vi "DelayPtsAdjust.vi"(7 "CalcPt?":bool=TRUE, 10 "Digitizer Settings":T1 {"Trigger Settings"."Trig Slope" items=["Positive", "Negative"]; "Trigger Settings"."Level (mV)" format="%.2f"; "Trigger Settings"."Trig Coupling" items=["DC 1 MOhm", "AC 1 MOhm", "DC 50 Ohm", "AC 50 Ohm"]; "Trigger Settings"."Trig Source" items=["Chan 1", "External"]; "Rel Dig Delay" format="%.2f"; "DigTimeOut" format="%.2f"; "Avg Num" min=1; "Offset delay (us)" format="%.2f"; "Additional dig delay (us)" format="%.2f"; "Digitizer delay (us)" format="%.2f"}, 11 "Delay in Pts":u32) -> (2 "Actual Delay pts":u32, 3 "PostDelayCorrection":u32)   [LabVIEW 2022 SP3]
uses:
  DigitizerSettings.ctl
  Digitizer.ctl
  DigConfig.ctl
  DigitizerID.ctl
  C:/Windows/System32/ADQAPI_dotNet_helper.dll
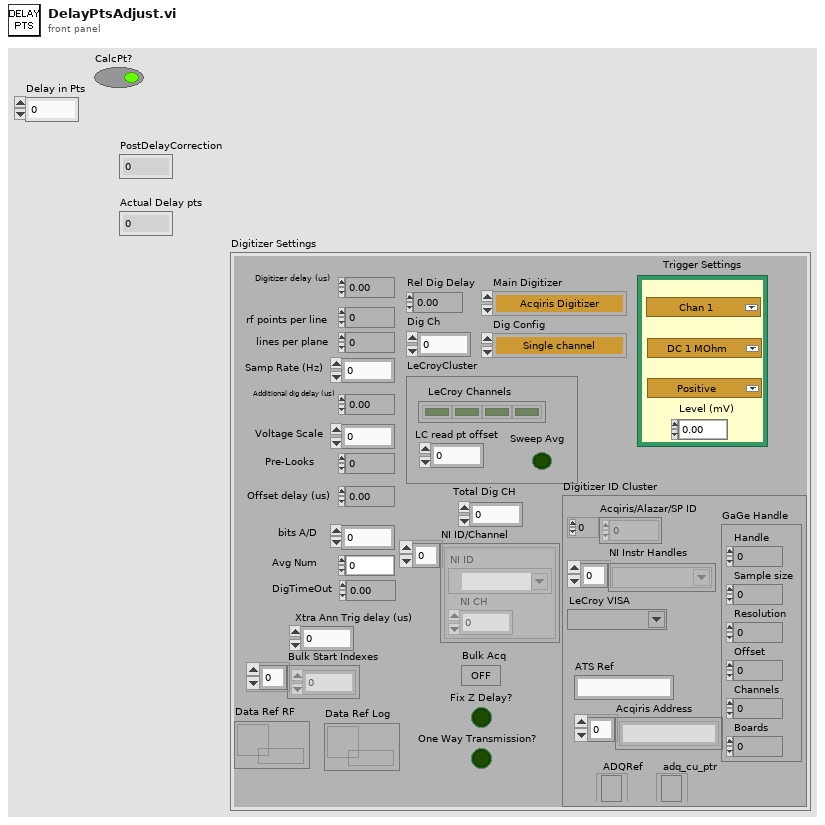
[diagram p1: front panel]
types:
  T1 = typedef "DigitizerSettings.ctl" = cluster{"Digitizer delay (us) ":dbl, "rf points per line":i32, "lines per plane":i32, "Samp Rate (Hz)":dbl, "Additional dig delay (us)":dbl, "Voltage Scale":dbl, "Pre-Looks":i32, "Offset delay (us)":dbl, "bits A/D":i8, "Avg Num":i32, "DigTimeOut":sgl, "Rel Dig Delay":sgl, "Dig Ch":i32, "LeCroyCluster":cluster{"LeCroy Channels":bool[], "LC read pt offset":dbl, "Sweep Avg":bool}, "Main Digitizer":T2, "Dig Config":T3, "Digitizer ID Cluster":T4, "Trigger Settings":cluster{"Trig Source":u16, "Trig Coupling":u16, "Trig Slope":u16, "Level (mV)":dbl}, "Bulk Acq":bool, "Bulk Start Indexes":i32[], "Data Ref RF":refnum<data-value>, "NI ID/Channel":cluster{"NI ID":refnum<k15>, "NI CH":i32}[], "Total Dig CH":i32, "Xtra Ann Trig delay (us)":dbl, "Fix Z Delay?":bool, "One Way Transmission?":bool, "Data Ref Log":refnum<data-value>}
  T2 = typedef "Digitizer.ctl" = enum16{"Acqiris Digitizer", "NI Digitizer", "LeCroy", "GaGe", "AlazarTech", "No Digitizer", "Teledyne"}
  T3 = typedef "DigConfig.ctl" = enum16{"Single channel", "2 Chans w/ 2 Acqiris", "2 Chans w/ 1 Acqiris", "5-CH Pulser New", "5-CH pulser w/ ann array", "5-pass style ann array", "Empty"}
  T4 = typedef "DigitizerID.ctl" = cluster{"Acqiris/Alazar/SP ID":u32[], "NI Instr Handles":refnum<k15>[], "LeCroy VISA":refnum<visa-resource-name>, "GaGe Handle":cluster{"Handle":u32, "Sample size":u32, "Resolution":i32, "Offset":i32, "Channels":u32, "Boards":u32}, "ATS Ref":string, "Acqiris Address":string[], "ADQRef":refnum<k24>, "adq_cu_ptr":refnum<k24>}
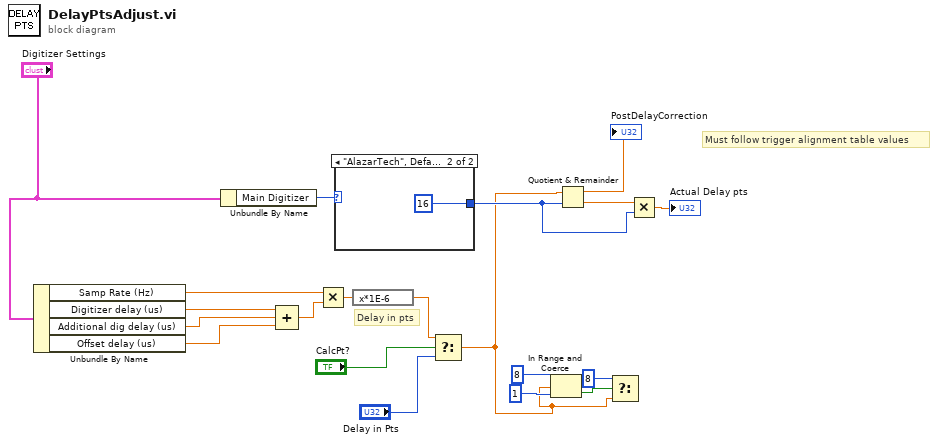
[diagram p0: block diagram]
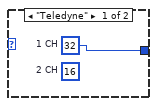
[diagram p2: hidden frame]
diagram:
  # "Delay in pts"
  # "Must follow trigger alignment table values"
  n1 = Unbundle By Name("Digitizer Settings") -> ("Samp Rate (Hz)"=w6:dbl, "Digitizer delay (us)"=w10:dbl, "Additional dig delay (us)"=w9:dbl, "Offset delay (us)"=w8:dbl)
  n2 = Unbundle By Name("Digitizer Settings") -> ("Main Digitizer"=w12:T2)
  n3 = Compound Arithmetic op=ADD(w10, w9, w8) -> (w7:dbl)
  n4 = Multiply(x=w6, y=w7) -> (x*y=w11:dbl)
  n5 = case shown="\"AlazarTech\", Default" w12 {
    tunnel: [w21 u32 16 ("upper limit")] -> w17
    frame "Teledyne" {
      (unwired) 16  # 2 CH
      w21 = 32  # 1 CH
    }
    frame "AlazarTech", Default {
    }
  }
  n6 = expression code="x*1E-6"(w11) -> (w4:dbl)
  n7 = Select(t=w4, s="CalcPt?", f="Delay in Pts") -> (s? t:f=w2:dbl)
  n8 = In Range and Coerce(upper limit=u32 8, x=w2, lower limit=u32 1) -> (In Range?=w13:bool)  [unwired: 1 out]
  n9 = Quotient & Remainder(x=w2, y=w17) -> (x-y*floor(x/y)=→"PostDelayCorrection":dbl, floor(x/y)=w18:dbl)
  n10 = Select(t=u32 8, s=w13, f=w2) -> ()  [unwired: 1 out]
  n11 = Multiply(x=w18, y=w17) -> (x*y=→"Actual Delay pts":dbl)
